vi "Write VI Interpreter.vi"(5 "VI Interpreter":refnum<class "VI Interpreter.lvclass">, 9 "RasPi Compiler in":refnum<class "RasPi Compiler.lvclass">) -> (3 "RasPi Compiler out":refnum<class "RasPi Compiler.lvclass">)   [LabVIEW 2014, in "RasPi Compiler.lvclass"]
uses:
  RasPi Compiler.lvclass
  VI Interpreter/Classes/VI Interpreter/VI Interpreter.lvclass
  RasPi Compiler.lvclass/RasPi Compiler.ctl
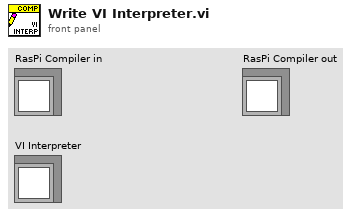
[diagram p1: front panel]
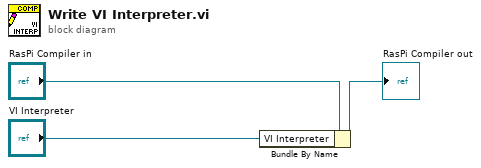
[diagram p0: block diagram]
diagram:
  n1 = Bundle By Name(cluster="RasPi Compiler in", "VI Interpreter"="VI Interpreter") -> (→"RasPi Compiler out":refnum<class "RasPi Compiler.lvclass">)
